vi "Create All Message Queues.vi"(8 "error in (no error)":errorcluster) -> (0 "error out":errorcluster, 3 "Message Queues out":T1)   [LabVIEW 2015, in "Message Queue.lvlib"]
doc: "This VI creates and initializes all the message queues for your application. If your application requires more than one message queue, right-click the \"Message Queues\" constant above and select Open Type Def. Add the new Message Queue(s) to the type definition, then initialize them in this VI."
uses:
  Message Queue.lvlib
  All Message Queues.ctl
  Message Cluster.ctl
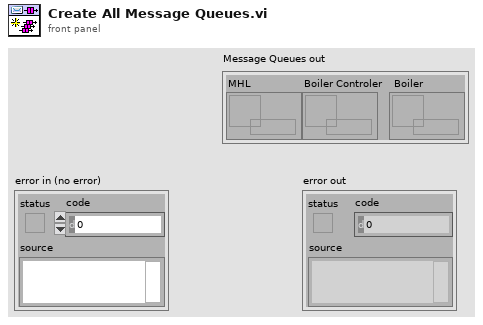
[diagram p1: front panel]
types:
  T1 = typedef "Message Queue.lvlib/All Message Queues.ctl" = cluster{"MHL":refnum<queue>, "Boiler Controler":refnum<queue>, " Boiler":refnum<queue>}
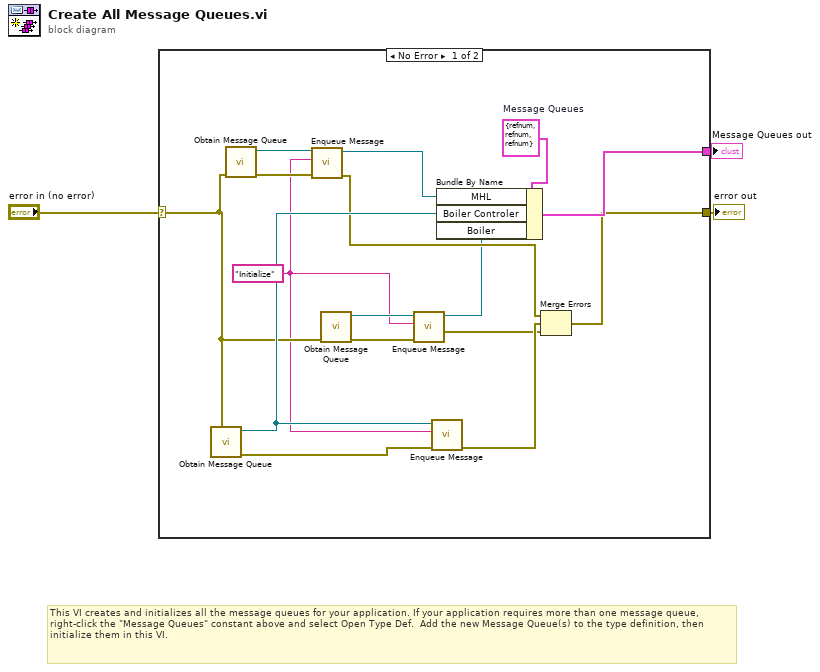
[diagram p0: block diagram]
diagram:
  # "This VI creates and initializes all the message queues for your application. If your application requires more than one message queue, right-click the \"Message Queues\" constant above and select Open Type Def.  Add the new Message Queue(s) to the type definition, then initialize them in this VI."
  n1 = case shown="No Error" "error in (no error)" {
    selector: "error in (no error)" -> [w7 w20]
    tunnel: [w10 w20] -> w3
    tunnel: [w18 _] -> w2
    frame No Error {
      w4 = "Initialize" ("Message")
      w19 = T1 {"MHL"=refnum, "Boiler Controler"=refnum, " Boiler"=refnum}  # Message Queues
      n2 = call "Obtain Message Queue.vi"("error in (no error)"=w7) -> ("error out"=w17:errorcluster, "Message Queue"=w14:refnum<queue>)  [unwired: 9 in]
      n3 = call "Obtain Message Queue.vi"("error in (no error)"=w7) -> ("error out"=w13:errorcluster, "Message Queue"=w16:refnum<queue>)  [unwired: 9 in]
      n4 = call "Enqueue Message.vi"("error in (no error)"=w13, "Message"=w4, "Message Queue"=w16) -> ("error out"=w12:errorcluster, "dup Message Queue"=w15:refnum<queue>)  [unwired: 7 in]
      n5 = call "Obtain Message Queue.vi"("error in (no error)"=w7) -> ("error out"=w8:errorcluster, "Message Queue"=w6:refnum<queue>)  [unwired: 9 in]
      n6 = call "Enqueue Message.vi"("error in (no error)"=w8, "Message"=w4, "Message Queue"=w6) -> ("error out"=w9:errorcluster, "dup Message Queue"=w5:refnum<queue>)  [unwired: 7 in]
      n7 = call "Enqueue Message.vi"("error in (no error)"=w17, "Message"=w4, "Message Queue"=w14) -> ("error out"=w11:errorcluster)  [unwired: 7 in, 1 out]
      n8 = Bundle By Name(cluster=w19, "MHL"=w15, "Boiler Controler"=w14, "Boiler"=w5) -> (w18:T1)
      n9 = Merge Errors(w12, w11, w9) -> (w10:errorcluster)
    }
    frame Error {
    }
  }
  "Message Queues out" <- w2
  "error out" <- w3
